vi "1D Rational Polynomial Evaluation (CDB).vi"(9 "A":cdb[](array[numeric]) format="%#.2f", 10 "Q(x)":cdb[](array[numeric]) format="%#.2f", 11 "P(x)":cdb[](array[numeric]) format="%#.2f") -> (0 "error":i32, 3 "P(A)/Q(A)":cdb[](array[numeric]))   [LabVIEW 2020, in "NI_AALPro.lvlib"]
doc: "Evaluates a rational polynomial at the points you specify in <B>A</B>. <B>P(x)</B> and <B>Q(x)</B> specify the numerator and denominator polynomial coefficients, respectively. The data types you wire to the <B>P(x)</B> and <B>Q(x)</B> inputs determine the polymorphic instance to use."
uses:
  NI_AALPro.lvlib
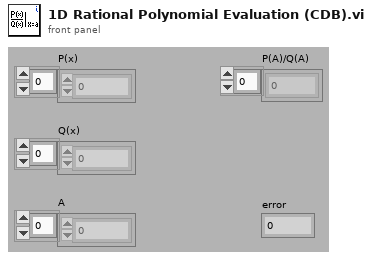
[diagram p1: front panel]
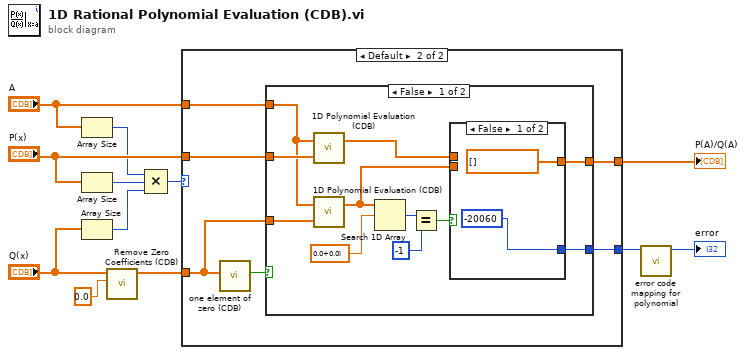
[diagram p0: block diagram]
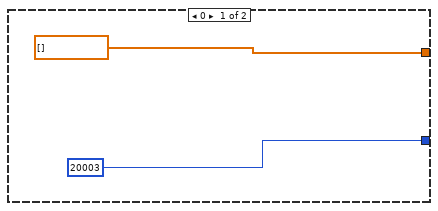
[diagram p2: hidden frame]
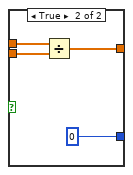
[diagram p3: hidden frame]
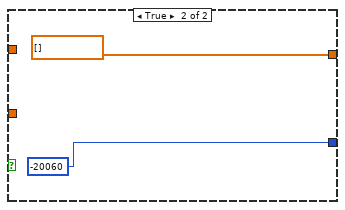
[diagram p4: hidden frame]
diagram:
  n1 = Array Size(array="A") -> (size(s)=w9:i32)
  n2 = Array Size(array="P(x)") -> (size(s)=w8:i32)
  n3 = Array Size(array="Q(x)") -> (size(s)=w7:i32)
  n4 = call "Remove Zero Coefficients (CDB).vi"("threshold"=0.0, "P(x) In"="Q(x)") -> ("P(x) Out"=w3:cdb[])  [unwired: 7 in, 2 out]
  n5 = Compound Arithmetic op=MULTIPLY(w9, w8, w7) -> (w6:i32)
  n6 = case shown="Default" w6 {
    tunnel: w3 -> [_ w17]
    tunnel: "P(x)" -> [_ w20]
    tunnel: "A" -> [_ w19]
    tunnel: [cdb[] [] w18] -> w12
    tunnel: [20003 ("empty array") w15] -> w2
    frame 0 {
    }
    frame Default {
      n7 = call "one element of zero (CDB).vi"("Array in"=w17) -> ("equal [0]?"=w16:bool)  [unwired: 10 in]
      n8 = case shown="False" w16 {
        tunnel: w20 -> [w30 _]
        tunnel: w19 -> [w29 _]
        tunnel: [w22 cdb[] [] ("CDB")] -> w18
        tunnel: w17 -> [w31 _]
        tunnel: [w21 -20060 ("divide by zero")] -> w15
        frame False {
          n9 = call "1D Polynomial Evaluation (CDB).vi"("P(x)"=w30, "A"=w29) -> ("P(A)"=w24:cdb[])  [unwired: 1 out]
          n10 = call "1D Polynomial Evaluation (CDB).vi"("P(x)"=w31, "A"=w29) -> ("P(A)"=w23:cdb[])  [unwired: 1 out]
          n11 = Search 1D Array(1D array=w23, element=cdb 0.0+0.0i) -> (index of element=w27:i32)  [unwired: 1 in]
          n12 = Equal?(x=w27, y=-1 ("empty array")) -> (x = y?=w25:bool)
          n13 = case shown="False" w25 {
            tunnel: w24 -> [_ w37]
            tunnel: w23 -> [_ w36]
            tunnel: [cdb[] [] ("CDB") w35] -> w22
            tunnel: [-20060 ("divide by zero") 0 ("empty array")] -> w21
            frame False {
            }
            frame True {
              n14 = Divide(x=w37, y=w36) -> (x/y=w35:cdb[])
            }
          }
        }
        frame True {
        }
      }
    }
  }
  "P(A)/Q(A)" <- w12
  n15 = call "error code mapping for polynomial.vi"("error in"=w2) -> ("error out"=→"error":i32)  [unwired: 10 in]
